vi "Periodic Messenger.vi"   [LabVIEW 2021]
uses:
  <vilib>/Platform/TimedLoop/XDataNode/timing_clust.ctl
  <vilib>/Platform/TimedLoop/XDataNode/nitl_modes.ctl
  <vilib>/Platform/TimedLoop/XDataNode/wakeup.ctl
  Type Definitions/Data Frame.ctl
  Type Definitions/Data Frame Header.ctl
  Type Definitions/Payload Class.ctl
  Type Definitions/Device.ctl
  <vilib>/platform/TimedLoop/XDataNode/XDataNode.xnode
  <vilib>/Platform/TimedLoop/XDataNode/XDNodeRunTimeDep.lvlib
types:
  T1 = typedef "XDNodeRunTimeDep.lvlib/timing_clust.ctl" = cluster{"Expected End [f-1]":u64, "Actual End [f-1]":u64, "Finished Late? [f-1]":bool, "Expected End [i-1]":u64, "Actual End [i-1]":u64, "Finished Late? [i-1]":bool, "Expected Start [i]":u64, "Actual Start [i]":u64, "Expected Start [f]":u64, "Actual Start [f]":u64, "Source Name":string, "Structure Name":string, "Period":i64, "Deadline":i64, "Offset":i64, "Start":i64, "Priority":i32, "Timeout":i32, "Mode":T2, "Wakeup Reason":T3, "Error":errorcluster, "Source Type":string, "Secondary Source Type":string, "Global End Time":u64, "Global Start Time":u64, "Frame Duration":u64, "Iteration Duration":u64, "Assigned CPU":i32, "I/O Scan Engine Mode":u32}
  T2 = typedef "XDNodeRunTimeDep.lvlib/nitl_modes.ctl" = enum32{"No Change", "Process missed periods, maintain original phase", "Discard missed periods, maintain original phase", "Process missed periods, ignore original phase", "Discard missed periods, ignore original phase"}
  T3 = typedef "XDNodeRunTimeDep.lvlib/wakeup.ctl" = enum32{"Normal", "Aborted", "Asynchronous wakeup", "Timing source error", "Timed loop error", "Timeout"}
  T4 = typedef "Data Frame.ctl" = cluster{"Frame Header":T5, "Payload":string, "CRC":u32}
  T5 = typedef "Data Frame Header.ctl" = cluster{"Sync":u32, "Time":dbl, "Nanosecond Counter":i64, "Payload Class":T6, "Payload ID":u16, "Counter":i32, "Options":u32, "Source":T7, "Destination":T7}
  T6 = typedef "Payload Class.ctl" = enum16{"System State", "Parameters", "Metadata", "Software Monitor", "Data", "Commands"}
  T7 = typedef "Device.ctl" = enum32{"None", "Exec", "Aux1", "Aux2", "Aux3"}
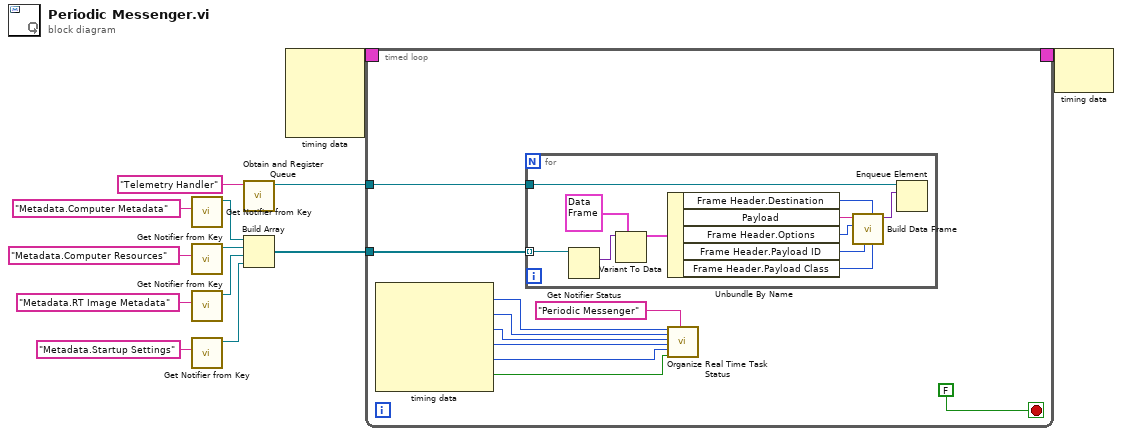
[diagram p0: block diagram]
diagram:
  n1 = call "Get Notifier from Key.vi"("Notifier Key"="Metadata.Computer Metadata") -> ("Notifier"=w3:refnum<notifier>)  [unwired: 8 in, 2 out]
  n2 = call "Get Notifier from Key.vi"("Notifier Key"="Metadata.Computer Resources") -> ("Notifier"=w5:refnum<notifier>)  [unwired: 8 in, 2 out]
  n3 = call "Get Notifier from Key.vi"("Notifier Key"="Metadata.RT Image Metadata") -> ("Notifier"=w8:refnum<notifier>)  [unwired: 8 in, 2 out]
  n4 = call "Get Notifier from Key.vi"("Notifier Key"="Metadata.Startup Settings") -> ("Notifier"=w9:refnum<notifier>)  [unwired: 8 in, 2 out]
  n5 = call "Obtain and Register Queue.vi"("Queue Name (unnamed)"="Telemetry Handler" ("name (unnamed)")) -> ("Queue Reference"=w11:refnum<queue>)  [unwired: 9 in, 1 out]
  n6 = Build Array(w3, w5, w8, w9) -> (w1:refnum<notifier>[])
  n7 = node-c288() -> (w13:T1)  [unwired: 4 in]
  n8 = timed-loop {
    timing: w13 -> [_]
    timing-out: [_] -> w12
    tunnel: w11 -> [w15]
    tunnel: w1 -> [w14]
    stop <- FALSE stop-if-true
    n9 = node-c288() -> (w21:i32, w20:i32, w19:i64, w18:i64, w17:i64, w16:bool)  [unwired: 1 in]
    n10 = for {
      tunnel: w14 -> [w34] mode=indexing
      tunnel: w15 -> [w33]
      n11 = Get Notifier Status(notifier=w34) -> (current notification=w30:variant)  [unwired: 1 in, 4 out]
      n12 = Variant To Data(type=T4 {"Frame Header"={"Sync"=0, "Time"=0.0, "Nanosecond Counter"=0, "Payload Class"=enum."System State", "Payload ID"=0, "Counter"=0, "Options"=0, "Source"=enum."None", "Destination"=enum."None"}, "Payload"="", "CRC"=0} ("Frame"), Variant=w30) -> (data=w31:T4)  [unwired: 1 in, 1 out]
      n13 = Unbundle By Name(w31) -> ("Frame Header.Destination"=w25:T7, "Payload"=w26:string, "Frame Header.Options"=w27:u32, "Frame Header.Payload ID"=w28:u16, "Frame Header.Payload Class"=w29:T6)
      n14 = call "Build Data Frame.vi"("Payload Class (Data)"=w29, "Destination (None)"=w25, "Payload ID (0)"=w28, "Options (0)"=w27, "Payload (Empty String)"=w26) -> ("Frame"=w24:variant)  [unwired: 5 in, 1 out]
      n15 = Enqueue Element(queue=w33, element=w24) -> ()  [unwired: 2 in, 3 out]
    }
    n16 = call "Organize Real Time Task Status.vi"("Priority"=w21, "Processor"=w20, "Offset"=w19, "Iteration Duration"=w18, "Period"=w17, "Finished Late? [i-1]"=w16, "Task Name"="Periodic Messenger") -> ()  [unwired: 12 in, 1 out]
  }
  n17 = node-c288(w12) -> ()  [unwired: 1 out]
